vi "Cryo Magnet (SubVI).vi"(0 "Instrument parameters":T1, 1 "String in":refnum<vi>, 3 "Max Rate":dbl=0.5 format="%#_13g", 5 "Target":dbl, 7 "Present value":dbl, 9 "Sweep rate":dbl, 11 "error in (no error)":errorcluster, 12 "Timeout (s)":u16, 14 "Default Rate":dbl=0.25 format="%#_13g") -> (4 "Instrument parameters out":T1, 6 "Last field":dbl, 15 "error out":errorcluster)   [LabVIEW 2025, in "Cryo.lvlib"]
uses:
  Cryo.lvlib
  TYPE DEFS/S2DS_Instrument parameters.ctl
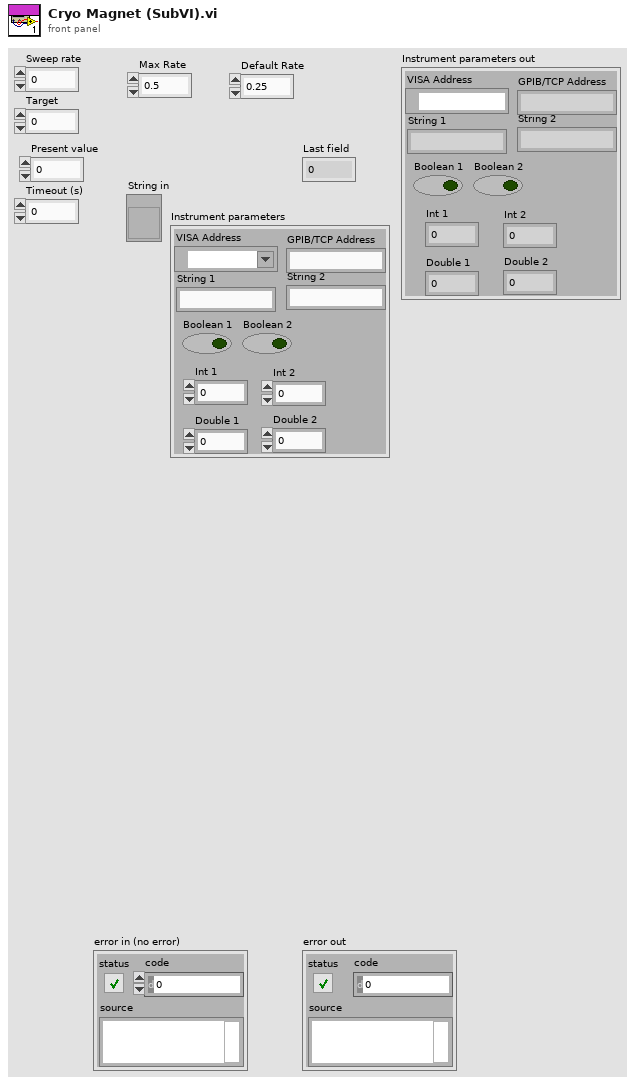
[diagram p1: front panel]
types:
  T1 = typedef "S2DS_Instrument parameters.ctl" = cluster{"VISA Address":refnum<visa-resource-name>, "GPIB/TCP Address":string, "String 1":string, "String 2":string, "Boolean 1":bool, "Boolean 2":bool, "Int 1":i32, "Int 2":i32, "Double 1":dbl, "Double 2":dbl}
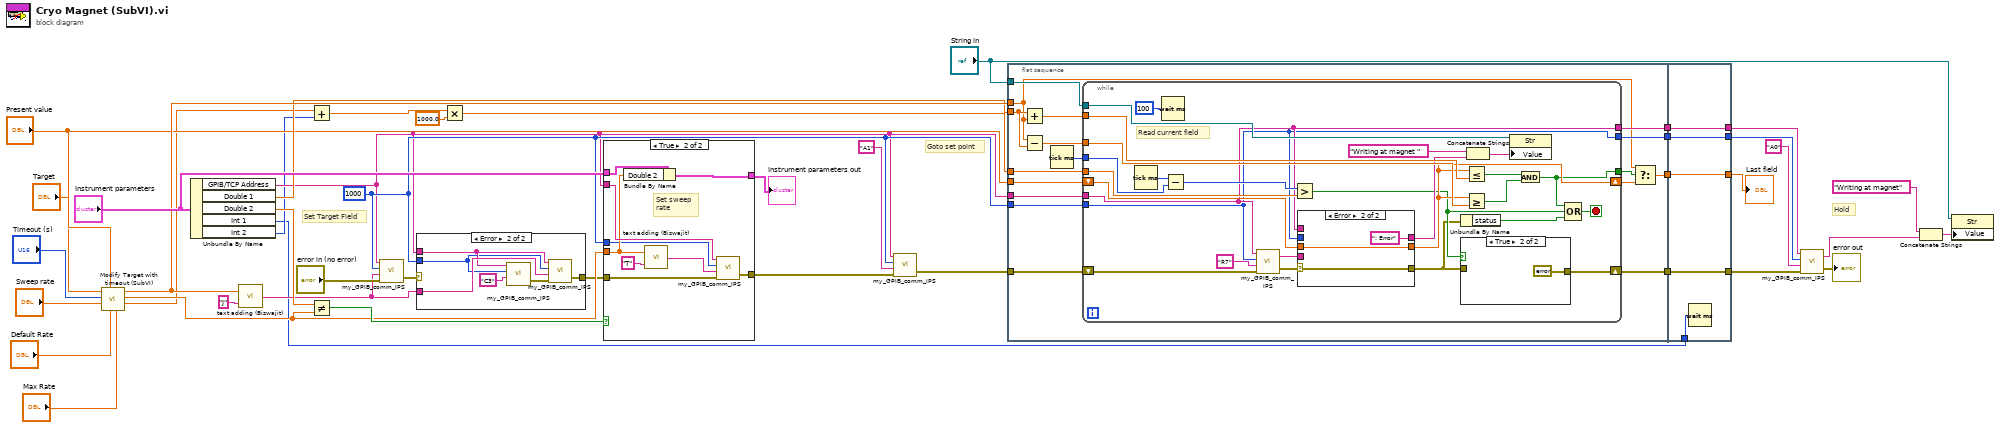
[diagram p0: block diagram]
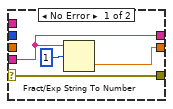
[diagram p4: hidden frame]
diagram:
  w6 = u32 1000 ("Timeout (ms)")
  # "Goto set point"
  # "Set Target Field"
  # "Hold"
  n1 = call "Modify Target with timeout (SubVI).vi"("Max Rate"="Max Rate", "Default Rate"="Default Rate", "Target in"="Target", "Sweep rate in"="Sweep rate", "Timeout (s) in"="Timeout (s)", "Present value"="Present value") -> ("Timeout (s) out"=w11:dbl, "Sweep rate out"=w15:dbl, "Target out"=w17:dbl)  [unwired: 3 in]
  n2 = Unbundle By Name("Instrument parameters") -> ("GPIB/TCP Address"=w4:string, "Double 1"=w13:dbl, "Double 2"=w20:dbl, "Int 1"=w1:i32, "Int 2"=w2:i32)
  n3 = call "text adding (Biswajit).vi"("string"="J", "number"=w17) -> ("String"=w5:string)
  n4 = Add(x=w11, y=w2) -> (x+y=w10:dbl)
  n5 = Not Equal?(x=w20, y=w15) -> (x != y?=w19:bool)
  n6 = call "my_GPIB_comm_IPS.vi"("error in"="error in (no error)", "Command"=w5, "Timeout (ms)"=w6, "GPIB address"=w4) -> ("error out"=w8:errorcluster)  [unwired: 1 out]
  n7 = case shown="Error" w8 {
    selector: w8 -> [w44 _]
    tunnel: [w44 w45] -> w7
    tunnel: w4 -> [_ w47]
    tunnel: w6 -> [_ w46]
    tunnel: w5 -> [_ w48]
    frame No Error {
    }
    frame Error {
      n8 = call "my_GPIB_comm_IPS.vi"("Command"="C3", "Timeout (ms)"=w46, "GPIB address"=w47) -> ("error out"=w49:errorcluster)  [unwired: 1 in, 1 out]
      n9 = call "my_GPIB_comm_IPS.vi"("error in"=w49, "Command"=w48, "Timeout (ms)"=w46, "GPIB address"=w47) -> ("error out"=w45:errorcluster)  [unwired: 1 out]
    }
  }
  n10 = Multiply(x=w10, y=1000.0) -> (x*y=w21:dbl)
  n11 = case shown="True" w19 {
    tunnel: w4 -> [_ w61]
    tunnel: w7 -> [w52 w60]
    tunnel: [w52 w59] -> w29
    tunnel: w15 -> [_ w55]
    tunnel: "Instrument parameters" -> [w51 w56]
    tunnel: w6 -> [_ w54]
    tunnel: [w51 w53] -> w3
    frame False {
    }
    frame True {
      # "Set sweep \nrate"
      n12 = Bundle By Name(cluster=w56, "Double 2"=w55) -> (w53:T1)
      n13 = call "text adding (Biswajit).vi"("string"="T", "number"=w55) -> ("String"=w58:string)
      n14 = call "my_GPIB_comm_IPS.vi"("error in"=w60, "Command"=w58, "Timeout (ms)"=w54, "GPIB address"=w61) -> ("error out"=w59:errorcluster)  [unwired: 1 out]
    }
  }
  "Instrument parameters out" <- w3
  n15 = call "my_GPIB_comm_IPS.vi"("error in"=w29, "Command"="A1", "Timeout (ms)"=w6, "GPIB address"=w4) -> ("error out"=w32:errorcluster)  [unwired: 1 out]
  n16 = flat-sequence {
    tunnel: w4 -> [w78]
    tunnel: w32 -> [w75]
    tunnel: w17 -> [w62]
    tunnel: w6 -> [w74]
    tunnel: w21 -> [w66]
    tunnel: w13 -> [w69]
    tunnel: [w77] -> w37
    tunnel: [w76] -> w36
    tunnel: [w63] -> w35
    tunnel: [w73] -> w34
    tunnel: "String in" -> [w71]
    tunnel: "Present value" -> [w67]
    tunnel: [w117] -> w31
    tunnel: [w119] -> w42
    tunnel: [w118] -> w33
    tunnel: w37 -> [w118]
    tunnel: w36 -> [w116]
    tunnel: w35 -> [w119]
    tunnel: w34 -> [w117]
    tunnel: [w116] -> w23
    tunnel: w1 -> [w115]
    frame #0 {
      n17 = Add(x=w69, y=w62) -> (x+y=w70:dbl)
      n18 = Subtract(x=w62, y=w69) -> (x-y=w68:dbl)
      n19 = Tick Count (ms)() -> (millisecond timer value=w72:u32)
      n20 = while {
        tunnel: w78 -> [w86]
        tunnel: [w86] -> w77
        shift-right: [w96] -> w76
        shift-left: w75 -> [w101]
        tunnel: w74 -> [w85]
        tunnel: [w85] -> w73
        tunnel: w72 -> [w99]
        tunnel: w66 -> [w97]
        tunnel: w71 -> [w95]
        tunnel: w70 -> [w91]
        tunnel: w68 -> [w90]
        shift-right: [w88] -> w64
        shift-left: w67 -> [w87]
        tunnel: [w79] -> w65
        stop <- w82 stop-if-true
        # "Read current field"
        n21 = Tick Count (ms)() -> (millisecond timer value=w100:u32)
        n22 = Wait (ms)(milliseconds to wait=u32 100) -> ()  [unwired: 1 out]
        n23 = Subtract(x=w100, y=w99) -> (x-y=w98:u32)
        n24 = call "my_GPIB_comm_IPS.vi"("error in"=w101, "Command"="R7", "Timeout (ms)"=w85, "GPIB address"=w86) -> ("error out"=w92:errorcluster, "Reply from Instrument"=w89:string)
        n25 = Greater?(x=w98, y=w97) -> (0:w83:bool)
        n26 = case shown="Error" w92 {
          selector: w92 -> [w107 w111]
          tunnel: w89 -> [w106 _]
          tunnel: [w108 w112] -> w88
          tunnel: w87 -> [_ w112]
          tunnel: w86 -> [_ _]
          tunnel: w85 -> [_ _]
          tunnel: [w107 w111] -> w81
          tunnel: [w106 ": Error" ("Reply from Instrument")] -> w84
          frame No Error {
            n27 = Fract/Exp String To Number(string=w106, offset=1) -> (number=w108:dbl)  [unwired: 3 out]
          }
          frame Error {
          }
        }
        n28 = Unbundle By Name(w81) -> ("status"=w80:bool)
        n29 = case shown="True" w83 {
          tunnel: [w113 errorcluster {"status"=TRUE, "code"=12345, "source"="Magnet timed out!!! "} ("error out")] -> w96
          tunnel: w81 -> [w113 _]
          frame False {
          }
          frame True {
          }
        }
        n30 = Less Or Equal?(x=w88, y=w91) -> (x <= y?=w104:bool)
        n31 = Greater Or Equal?(x=w88, y=w90) -> (x >= y?=w103:bool)
        n32 = Concatenate Strings("Writing at magnet " ("string"), w84) -> (w93:string)
        n33 = property on="Property Node" class="Str"(reference=w95, "Value"=w93) -> ()  [unwired: 1 in, 2 out]
        n34 = And(x=w104, y=w103) -> (x .and. y?=w79:bool)
        n35 = Compound Arithmetic op=OR(w79, w83, w80) -> (w82:bool)
      }
      n36 = Select(t=w62, s=w65, f=w64) -> (s? t:f=w63:dbl)
    }
    frame #1 {
      n37 = Wait (ms)(milliseconds to wait=w115) -> ()  [unwired: 1 out]
    }
  }
  n38 = call "my_GPIB_comm_IPS.vi"("error in"=w23, "Command"="A0", "Timeout (ms)"=w31, "GPIB address"=w33) -> ("error out"=→"error out":errorcluster, "Reply from Instrument"=w25:string)
  n39 = Concatenate Strings("Writing at magnet" ("string"), w25) -> (w24:string)
  n40 = property on="Property Node" class="Str"(reference="String in", "Value"=w24) -> ()  [unwired: 1 in, 2 out]
  "Last field" <- w42
